vi "Read write Master.vi"(8 "error in (no error)":errorcluster, 10 "Modbus data unit in":refnum<class "Modbus Data Unit.lvclass">, 11 "Modbus master in":refnum<class "Network Master.lvclass">) -> (0 "error out":errorcluster, 1 "PDU valid?":bool, 2 "Modbus data unit out":refnum<class "Modbus Data Unit.lvclass">, 3 "Modbus master out":refnum<class "Network Master.lvclass">)   [LabVIEW 2021, in "Network Master.lvclass"]
doc: "This VI allows a mutex for the master API without restricting any other functions. This mutex is currently unimplemented."
uses:
  Network Master.lvclass
  Modbus Data Unit/Modbus Data Unit.lvclass
  Network Master.lvclass/Network Master.ctl
  Transmission Data Unit/Transmission Data Unit.lvclass
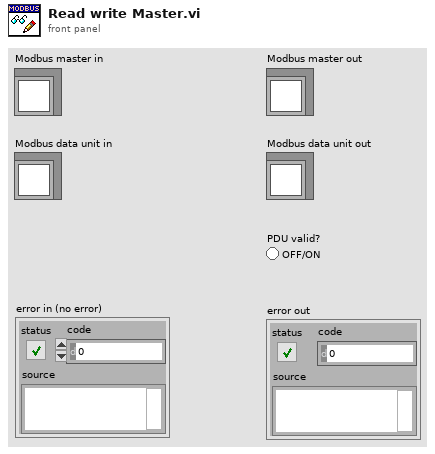
[diagram p1: front panel]
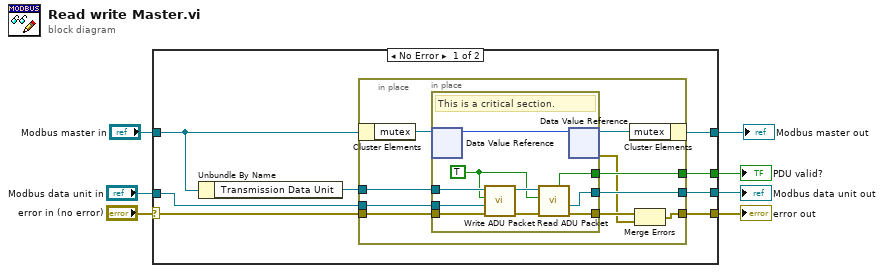
[diagram p0: block diagram]
diagram:
  n1 = case shown="No Error" "error in (no error)" {
    selector: "error in (no error)" -> [w10 w36]
    tunnel: "Modbus master in" -> [w9 w37]
    tunnel: [w15 w37] -> w6
    tunnel: "Modbus data unit in" -> [w14 w38]
    tunnel: [w13 w38] -> w4
    tunnel: [w12 w36] -> w3
    tunnel: [w11 _] -> w2
    frame No Error {
      n2 = Unbundle By Name(w9) -> ("Transmission Data Unit"=w8:refnum<class "Transmission Data Unit.lvclass">)
      n3 = in-place {
        in-place-border: w10 -> [w24]
        in-place-border: w14 -> [w23]
        in-place-border: [w21] -> w13
        in-place-border: [w20] -> w12
        in-place-border: [w19] -> w11
        in-place-border: w8 -> [w16]
        n4 = in-place-cluster #1(w9) -> ("mutex"=w25:refnum<data-value>)
        n5 = in-place {
          in-place-border: w24 -> [w32]
          in-place-border: w23 -> [w31]
          in-place-border: [w30] -> w18
          in-place-border: [w29] -> w21
          in-place-border: [w28] -> w19
          in-place-border: w16 -> [w27]
          w26 = TRUE ("isMaster (f)")
          # "This is a critical section."
          n6 = in-place-dvr #2(w25) -> (w33:u8)  [unwired: 1 out]
          n7 = call-dynamic "Write ADU Packet.vi"("error in"=w32, "modbus data unit"=w31, "isMaster (f)"=w26, "transmission data unit in"=w27) -> ("error out"=w35:errorcluster, "transmission data unit out"=w34:refnum<class "Transmission Data Unit.lvclass">)  [unwired: 6 in]
          n8 = call-dynamic "Read ADU Packet.vi"("error in"=w35, "isMaster (f)"=w26, "transmission data unit in"=w34) -> ("error out"=w30:errorcluster, "modbus data unit"=w29:refnum<class "Modbus Data Unit.lvclass">, "PDU Valid?"=w28:bool)  [unwired: 5 in, 1 out]
          n9 = in-place-dvr #2(w33) -> (w22:refnum<data-value>, w17:errorcluster)
        }
        n10 = in-place-cluster #1("mutex"=w22) -> (w15:refnum<class "Network Master.lvclass">)
        n11 = Merge Errors(w18, w17) -> (w20:errorcluster)
      }
    }
    frame Error {
    }
  }
  "Modbus data unit out" <- w4
  "Modbus master out" <- w6
  "error out" <- w3
  "PDU valid?" <- w2
